vi "Handle Response.vi"(7 "Inputs":T2, 8 "error in (no error)":errorcluster, 11 "Session Response Handler in":refnum<class "Session Response Handler.lvclass">) -> (0 "error out":errorcluster, 5 "Outputs":T1)   [LabVIEW 2020, in "HTTP Server.lvlib" / "Session Response Handler.lvclass"]
uses:
  Session Response Handler.lvclass
  Session Response Handler.lvclass/Session Response Handler.ctl
  Arguments/Arguments.lvclass
  <vilib>/IlluminatedG/IG HTTP Utils/HTTP Utils/Request/Request.lvclass
  <vilib>/IlluminatedG/IG HTTP Utils/HTTP Utils/Response/Response.lvclass
  Session/Session.lvclass
  Response Inputs.ctl
  HTTP Server.lvlib
  Response Outputs.ctl
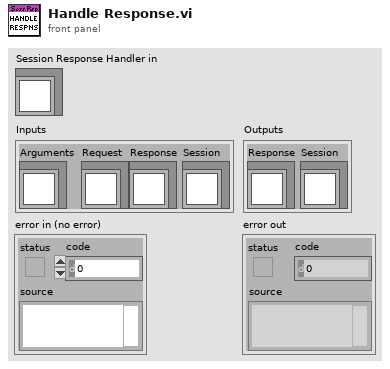
[diagram p1: front panel]
types:
  T1 = typedef "HTTP Server.lvlib/Response Outputs.ctl" = cluster{"Response":refnum<class "Response.lvclass">, "Session":refnum<class "Session.lvclass">}
  T2 = typedef "HTTP Server.lvlib/Response Inputs.ctl" = cluster{"Arguments":refnum<class "Arguments.lvclass">, "Request":refnum<class "Request.lvclass">, "Response":refnum<class "Response.lvclass">, "Session":refnum<class "Session.lvclass">}
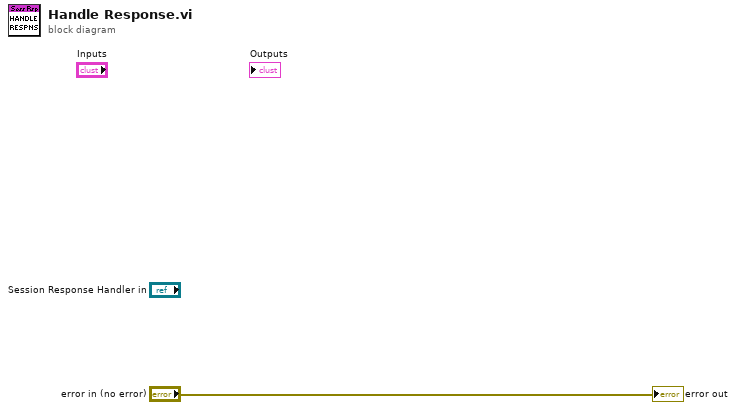
[diagram p0: block diagram]
diagram:
  "error out" <- "error in (no error)"
